vi "tls library paths.vi"() -> (0 "libssl":path=path "C:/Users/IEUser/Desktop/tlssimple/lvlibtls/libssl-43.dll", 1 "libcrypto":path=path "C:/Users/IEUser/Desktop/tlssimple/lvlibtls/libcrypto-41.dll", 2 "libtls":path=path "C:/Users/IEUser/Desktop/tlssimple/lvlibtls/libtls-15.dll", 3 "lvtls":path=path "C:/Users/IEUser/Desktop/tlssimple/lvlibtls/lvlibtls.dll")   [LabVIEW 2016, in "lv tls dll.lvlib"]
uses:
  lv tls dll.lvlib
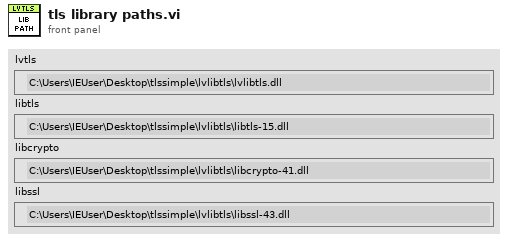
[diagram p1: front panel]
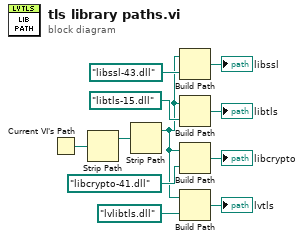
[diagram p0: block diagram]
diagram:
  n1 = Current VI's Path() -> (path=w11:path)
  n2 = Strip Path(path=w11) -> (stripped path=w2:path)  [unwired: 1 out]
  n3 = Strip Path(path=w2) -> (stripped path=w1:path)  [unwired: 1 out]
  n4 = Build Path(base path=w1, name or relative path=path "libssl-43.dll" ("libtls")) -> (appended path=→"libssl":path)
  n5 = Build Path(base path=w1, name or relative path=path "libtls-15.dll" ("libtls")) -> (appended path=→"libtls":path)
  n6 = Build Path(base path=w1, name or relative path=path "libcrypto-41.dll" ("libtls")) -> (appended path=→"libcrypto":path)
  n7 = Build Path(base path=w1, name or relative path=path "lvlibtls.dll" ("lvtls")) -> (appended path=→"lvtls":path)
